vi "Scope_V1_BK.vi"() -> ()   [LabVIEW 2011]
panel:
  out "波形图表":dbl(graph)
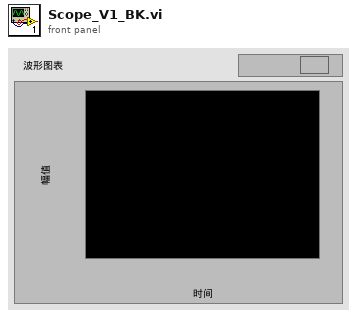
[diagram p1: front panel]
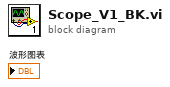
[diagram p0: block diagram]
diagram:
